vi "Transcriptor LabVIEW to C code 1.vi"(8 "error in (no error)":errorcluster, 9 "nested level":i32, 10 "GObject stop":refnum<vi>, 11 "GObject start":refnum<vi>) -> (0 "error out":errorcluster, 3 "Transcripted code":string)   [LabVIEW 2014]
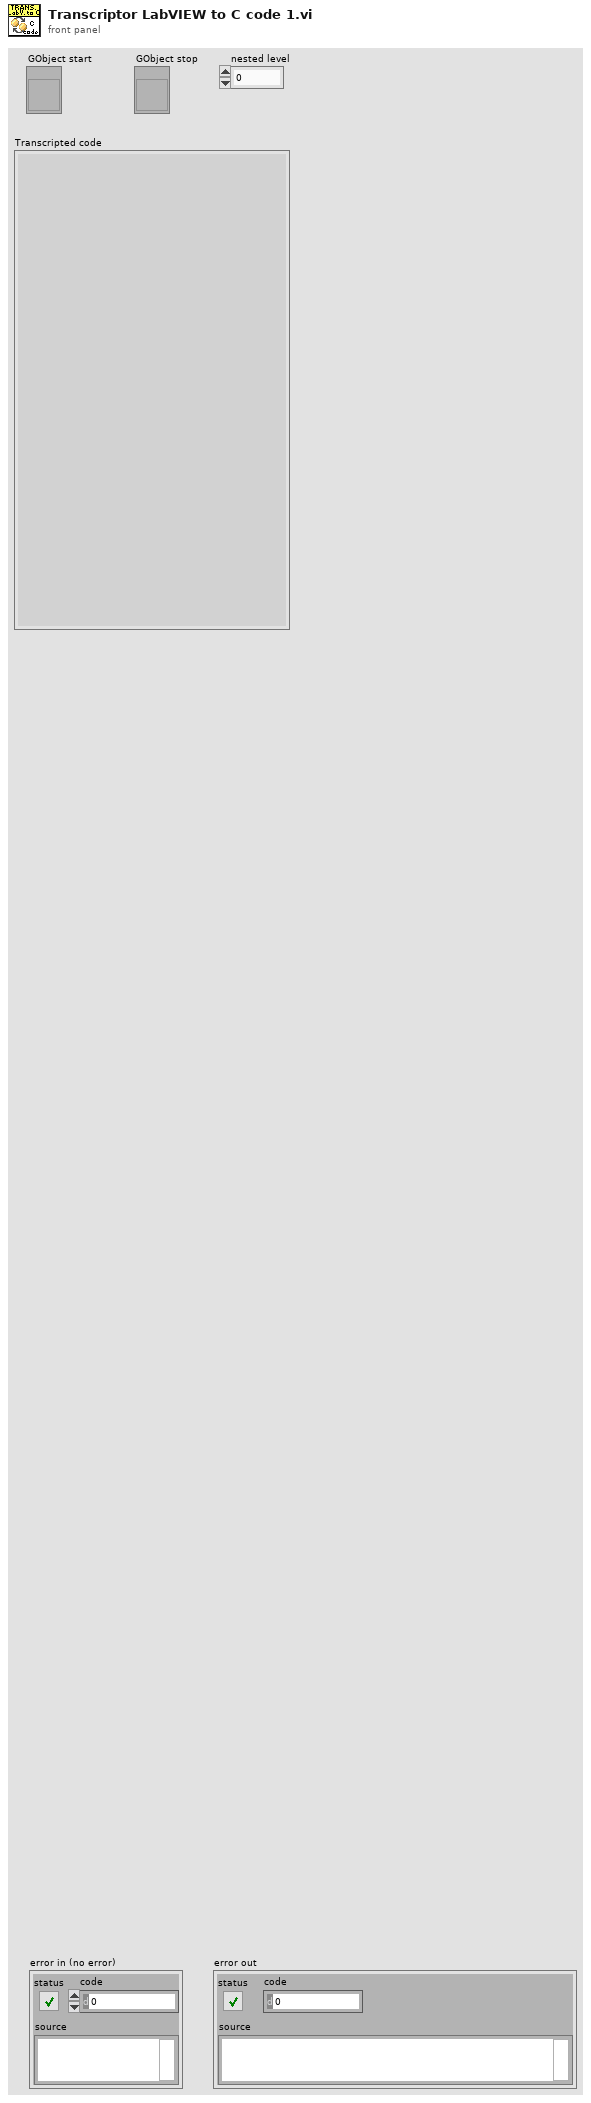
[diagram p1: front panel]
types:
  T1 = cluster{"transcripted code":string[], "element translation order":string[]}
  T2 = cluster{"terminals datatypes":string[][], "terminal\nconnected?":bool[], "terminal captions":string[], "term. count":i32, "terminal\nIsSource?":bool[], "SubVI name":string, "connected\nwires refs.":refnum<vi>[], "coerced\ndot?":bool[], "terminals[]":refnum<vi>[]}
  T3 = cluster{"terminals datatypes":string[][], "terminal\nconnected?":bool[], "terminal captions":string[], "term. count":i32, "terminal\nIsSource?":bool[], "SubVI name":string, "connected\nwires refs.":refnum<vi>[], "coerced dot?":bool[], "terminals[]":refnum<vi>[]}
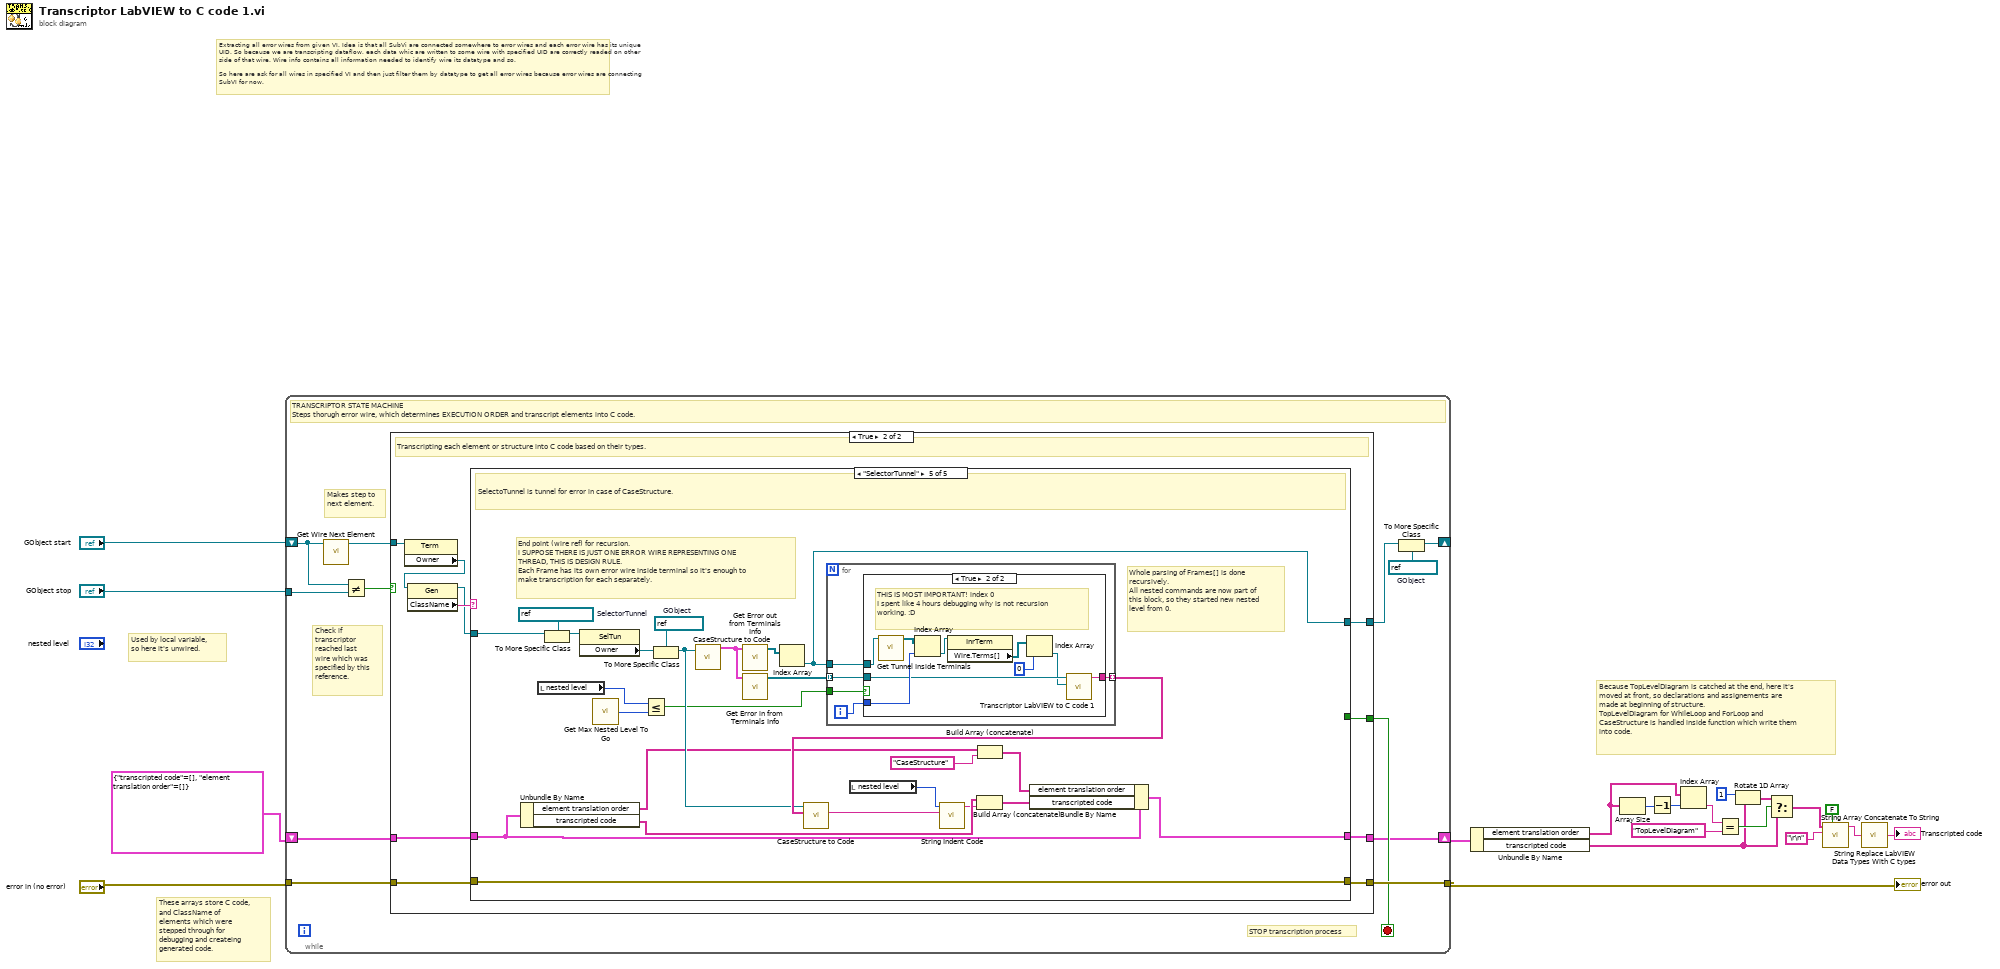
[diagram p0: block diagram]
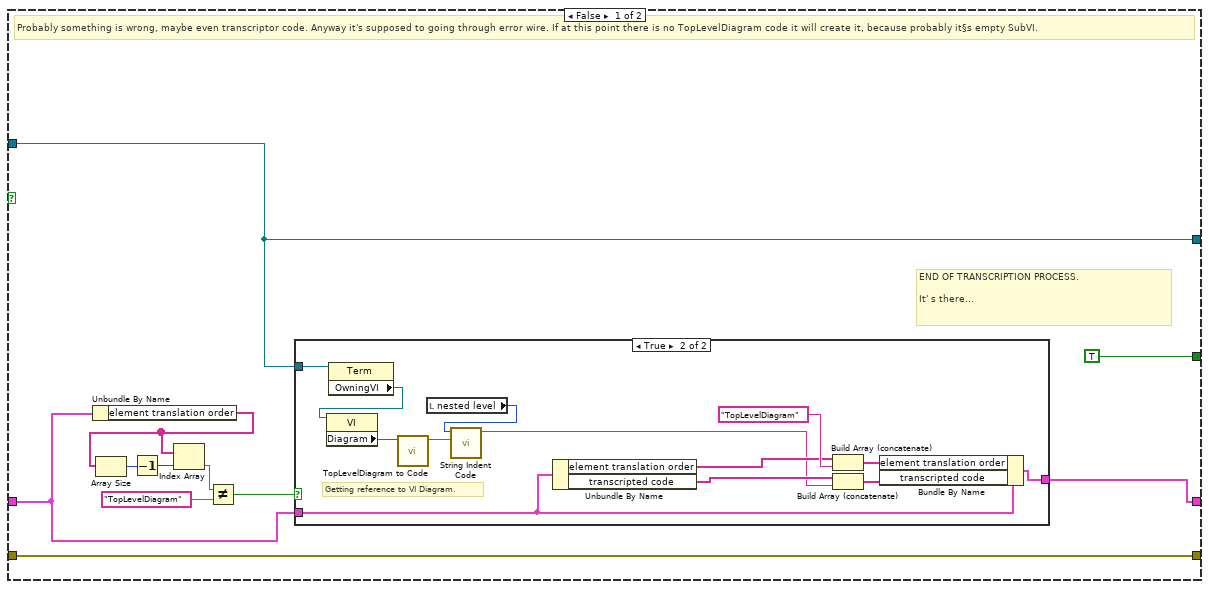
[diagram p2: hidden frame]
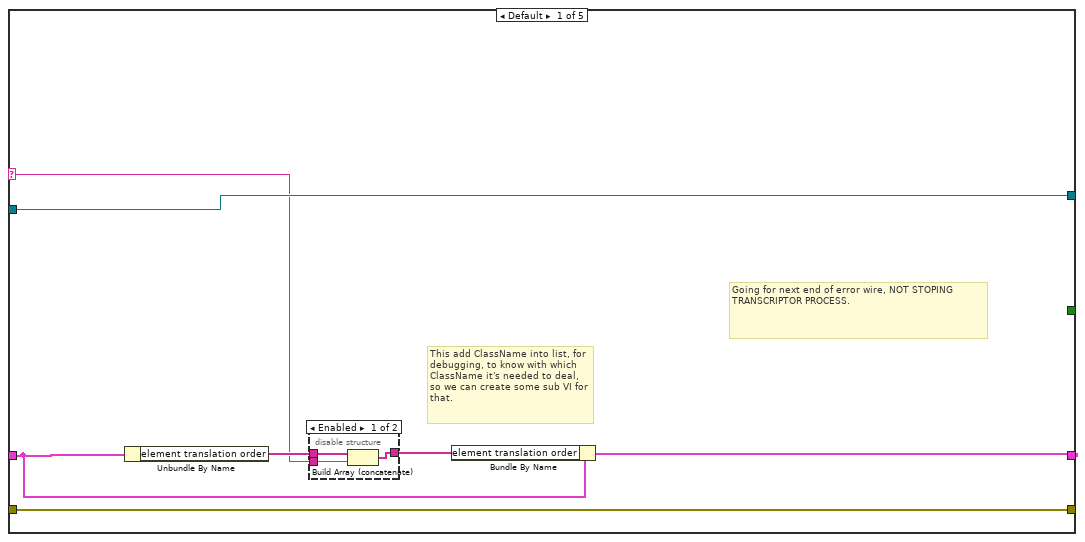
[diagram p4: hidden frame]
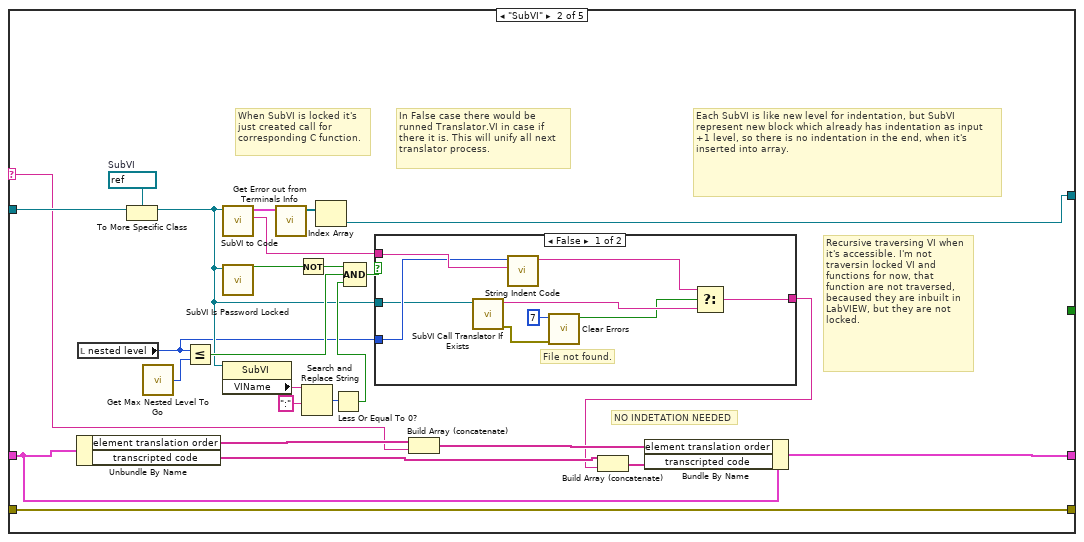
[diagram p6: hidden frame]
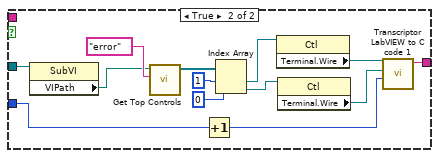
[diagram p7: hidden frame]
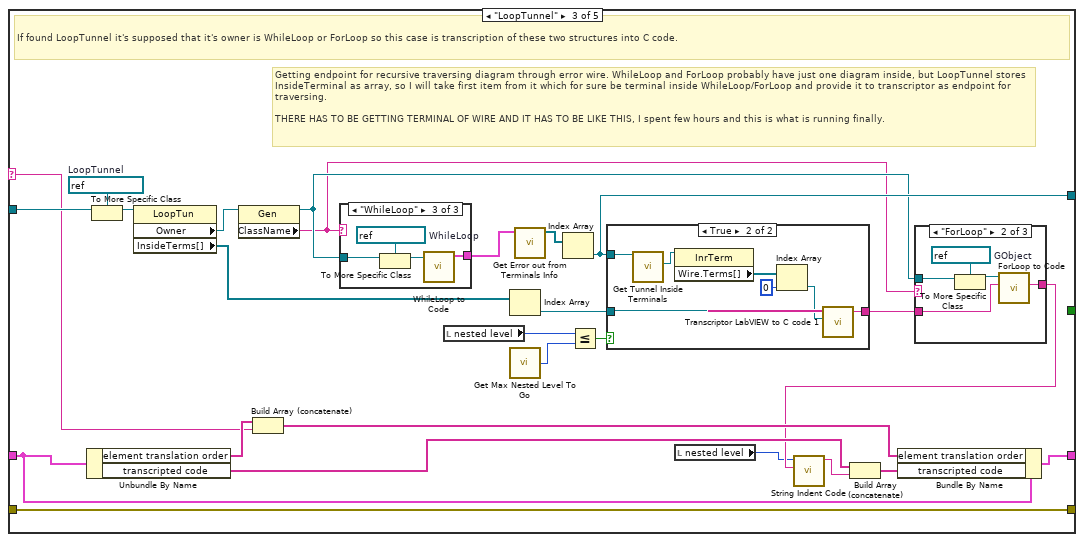
[diagram p8: hidden frame]
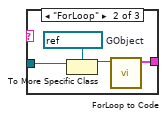
[diagram p10: hidden frame]
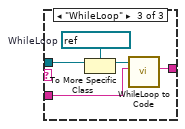
[diagram p12: hidden frame]
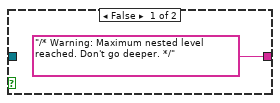
[diagram p13: hidden frame]
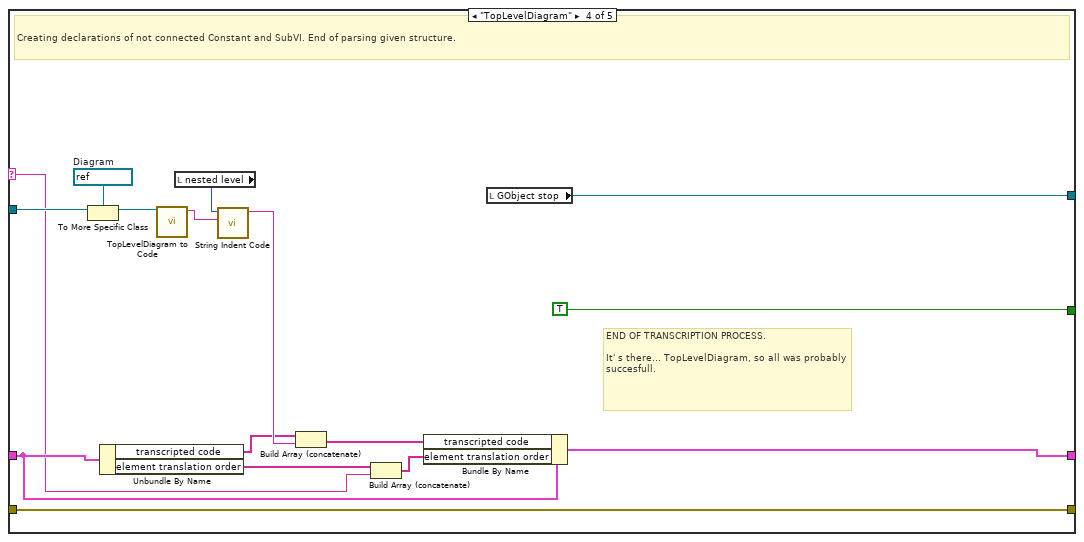
[diagram p14: hidden frame]
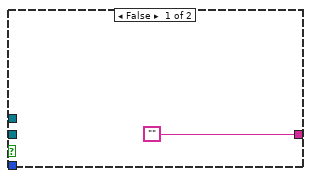
[diagram p15: hidden frame]
diagram:
  # "Because TopLevelDiagram is catched at the end, here it's moved at front, so declarations and assignements are made at beginning of structure.\nTopLevelDiagram for WhileLoop and ForLoop and CaseStructure is handled inside function which write them into code."
  # "Used by local variable, so here it's unwired."
  # "These arrays store C code, and ClassName of elements which were stepped through for debugging and createing generated code."
  # "Extracting all error wires from given VI. Idea is that all SubVi are connected somewhere to error wires and each error wire has its unique UID. So because we are transcripting dataflow, each data whic are written to some wire with specified UID are correctly readed on other side of that wire. Wire info contains all information needed to identify wire its datatype and so.\n\nSo here are ask for all wires in specified VI and then just filter them by datatype to get all error wires because error wires are connecting SubVI for now."
  n1 = while {
    tunnel: [w31] -> w15
    tunnel: "error in (no error)" -> [w30]
    shift-right: [w26] -> _
    shift-left: "GObject start" -> [w22]
    tunnel: "GObject stop" -> [w21]
    shift-right: [w24] -> w16
    shift-left: T1 {"transcripted code"=[], "element translation order"=[]} -> [w25]
    stop <- w29 stop-if-true
    w28 = refnum<vi> refnum  # GObject
    # "Makes step to next element."
    # "Check if transcriptor reached last wire which was specified by this reference."
    # "STOP transcription process"
    # "TRANSCRIPTOR STATE MACHINE\nSteps thorugh error wire, which determines EXECUTION ORDER and transcript elements into C code."
    n2 = call "Get Wire Next Element.vi"("start object"=w22) -> ("next terminal"=w32:refnum<vi>)  [unwired: 9 in, 1 out]
    n3 = Not Equal?(x=w22, y=w21) -> (x != y?=w23:bool)
    n4 = case shown="True" w23 {
      tunnel: w32 -> [w35 w63]
      tunnel: [w43 w67] -> w31
      tunnel: w30 -> [w43 w66]
      tunnel: [w35 w65] -> w27
      tunnel: [TRUE w64] -> w29
      tunnel: w25 -> [w34 w62]
      tunnel: [w33 w61] -> w24
      frame False {
        # "END OF TRANSCRIPTION PROCESS.\n\nIt' s there..."
        # "Probably something is wrong, maybe even transcriptor code. Anyway it's supposed to going through error wire. If at this point there is no TopLevelDiagram code it will create it, because probably it§s empty SubVI."
        n5 = Unbundle By Name(w34) -> ("element translation order"=w41:string[])
        n6 = Array Size(array=w41) -> (size(s)=w40:i32)
        n7 = Decrement(x=w40) -> (x-1=w39:i32)
        n8 = Index Array(array=w41, index=w39) -> (element=w38:string)
        n9 = Not Equal?(x=w38, y="TopLevelDiagram") -> (x != y?=w36:bool)
        n10 = case shown="True" w36 {
          tunnel: w35 -> [_ w57]
          tunnel: w34 -> [w44 w51]
          tunnel: [w44 w52] -> w33
          frame False {
          }
          frame True {
            # "Getting reference to VI Diagram."
            n11 = property class="Term"(reference=w57) -> ("OwningVI"=w54:refnum<vi>)  [unwired: 1 in, 2 out]
            n12 = property class="VI"(reference=w54) -> ("Diagram"=w53:refnum<vi>)  [unwired: 1 in, 2 out]
            n13 = call "TopLevelDiagram to Code.vi"("Diagram ref"=w53) -> ("transcripted code"=w55:string)  [unwired: 10 in]
            n14 = local read "nested level"() -> (w56:i32)
            n15 = call "String Indent Code.vi"("complete code"=w55, "actual nested level"=w56) -> ("indented code"=w45:string)  [unwired: 9 in]
            n16 = Unbundle By Name(w51) -> ("element translation order"=w48:string[], "transcripted code"=w47:string[])
            n17 = Build Array (concatenate)(w48, "TopLevelDiagram" ("y")) -> (w49:string[])
            n18 = Build Array (concatenate)(w47, w45) -> (w46:string[])
            n19 = Bundle By Name(cluster=w51, "element translation order"=w49, "transcripted code"=w46) -> (w52:T1)
          }
        }
      }
      frame True {
        # "Transcripting each element or structure into C code based on their types."
        n20 = property class="Term"(reference=w63) -> ("Owner"=w59:refnum<vi>)  [unwired: 1 in, 2 out]
        n21 = property class="Gen"(reference=w59) -> (reference out=w58:refnum<vi>, "ClassName"=w60:string)  [unwired: 1 in, 1 out]
        n22 = case shown="\"SelectorTunnel\"" w60 {
          selector: w60 -> [w68 w79 w127 w179 _]
          tunnel: w58 -> [w73 w93 w151 w186 w216]
          tunnel: [w74 w103 w149 w194 w218] -> w67
          tunnel: w66 -> [w74 w103 w149 w194 w218]
          tunnel: [w73 w94 w144 w188 w208] -> w65
          tunnel: [_ _ _ TRUE _] -> w64
          tunnel: w62 -> [w71 w100 w142 w191 w203]
          tunnel: [w69 w99 w141 w190 w204] -> w61
          frame Default {
            # "Going for next end of error wire, NOT STOPING TRANSCRIPTOR PROCESS."
            # "This add ClassName into list, for debugging, to know with which ClassName it's needed to deal, so we can create some sub VI for that."
            n23 = Unbundle By Name(w71) -> ("element translation order"=w72:string[])
            n24 = disable-structure shown="Enabled" {
              disable-tunnel: w72 -> [w77 w78]
              disable-tunnel: w68 -> [w76 _]
              disable-tunnel: [w75 w78] -> w70
              frame Enabled {
                n25 = Build Array (concatenate)(w77, w76) -> (w75:string[])
              }
              frame Disabled {
              }
            }
            n26 = Bundle By Name(cluster=w71, "element translation order"=w70) -> (w69:T1)
          }
          frame "SubVI" {
            w104 = refnum<vi> refnum  # SubVI
            # "In False case there would be runned Translator.VI in case if there it is. This will unify all next translator process."
            # "When SubVI is locked it's just created call for corresponding C function."
            # "NO INDETATION NEEDED"
            # "Each SubVI is like new level for indentation, but SubVI represent new block which already has indentation as input +1 level, so there is no indentation in the end, when it's inserted into array."
            # "Recursive traversing VI when it's accessible. I'm not traversin locked VI and\nfunctions for now, that function are not traversed, becaused they are inbuilt in LabVIEW, but they are not locked."
            n27 = Unbundle By Name(w100) -> ("element translation order"=w96:string[], "transcripted code"=w97:string[])
            n28 = local read "nested level"() -> (w81:i32)
            n29 = To More Specific Class(target class=w104, reference=w93) -> (specific class reference=w83:refnum<vi>)  [unwired: 1 in, 1 out]
            n30 = call "Get Max Nested Level To Go.vi"() -> ("max nested level"=w82:i32)
            n31 = Less Or Equal?(x=w81, y=w82) -> (x <= y?=w90:bool)
            n32 = call "SubVI to Code.vi"("reference"=w83) -> ("C code"=w92:string, "SubVI terminals info"=w101:T2)  [unwired: 9 in]
            n33 = call "SubVI Is Password Locked.vi"("SubVI ref"=w83) -> ("isPasswordLocked?"=w89:bool)  [unwired: 9 in, 1 out]
            n34 = property class="SubVI"(reference=w83) -> ("VIName"=w87:string)  [unwired: 1 in, 2 out]
            n35 = call "Get Error out from Terminals Info.vi"("terminals info"=w101) -> ("error out terminals"=w102:refnum<vi>[])  [unwired: 9 in, 1 out]
            n36 = Not(x=w89) -> (.not. x?=w88:bool)
            n37 = Search and Replace String(input string=w87, search string=":") -> (number of replacements=w85:i32)  [unwired: 6 in, 3 out]
            n38 = Index Array(array=w102) -> (element=w94:refnum<vi>)  [unwired: 1 in]
            n39 = Less Or Equal To 0?(x=w85) -> (x <= 0?=w84:bool)
            n40 = Compound Arithmetic op=AND(w88, w90, w84) -> (w91:bool)
            n41 = case shown="False" w91 {
              tunnel: w83 -> [w110 w126]
              tunnel: [w112 w125] -> w80
              tunnel: w92 -> [w113 _]
              tunnel: w81 -> [w111 w124]
              frame False {
                # "File not found."
                n42 = call "SubVI Call Translator If Exists.vi"("SubVI Refnum"=w110) -> ("Error Out"=w109:errorcluster, "Replaced Code"=w107:string)  [unwired: 9 in]
                n43 = call "String Indent Code.vi"("complete code"=w113, "actual nested level"=w111) -> ("indented code"=w105:string)  [unwired: 9 in]
                n44 = call <vilib>:"Clear Errors.vi"("error in (no error)"=w109, "specific error code to clear (0: all)"=7) -> ("specific error cleared?"=w106:bool)  [unwired: 4 in, 1 out]
                n45 = Select(t=w105, s=w106, f=w107) -> (s? t:f=w112:string)
              }
              frame True {
                n46 = property class="SubVI"(reference=w126) -> ("VIPath"=w119:path)  [unwired: 1 in, 2 out]
                n47 = call "Get Top Controls.vi"("DataType"="error", "vi path"=w119) -> ("Controls Referencies Array"=w122:refnum<vi>[])  [unwired: 8 in, 1 out]
                n48 = Increment(x=w124) -> (x+1=w114:i32)
                n49 = Index Array(array=w122, index #1=1 ("index"), index #2=0 ("index")) -> (element #1=w118:refnum<vi>, element #2=w117:refnum<vi>)
                n50 = property on="Property Node" class="Ctl"(reference=w118) -> ("Terminal.Wire"=w116:refnum<vi>)  [unwired: 1 in, 2 out]
                n51 = property on="Property Node" class="Ctl"(reference=w117) -> ("Terminal.Wire"=w115:refnum<vi>)  [unwired: 1 in, 2 out]
                n52 = call "Transcriptor LabVIEW to C code 1.vi"("nested level"=w114, "GObject stop"=w115, "GObject start"=w116) -> ("Transcripted code"=w125:string)  [unwired: 7 in, 1 out]
              }
            }
            n53 = Build Array (concatenate)(w96, w79) -> (w95:string[])
            n54 = Build Array (concatenate)(w97, w80) -> (w98:string[])
            n55 = Bundle By Name(cluster=w100, "element translation order"=w95, "transcripted code"=w98) -> (w99:T1)
          }
          frame "LoopTunnel" {
            w152 = refnum<vi> refnum  # LoopTunnel
            # "Getting endpoint for recursive traversing diagram through error wire. WhileLoop and ForLoop probably have just one diagram inside, but LoopTunnel stores InsideTerminal as array, so I will take first item from it which for sure be terminal inside WhileLoop/ForLoop and provide it to transcriptor as endpoint for traversing.\n\nTHERE HAS TO BE GETTING TERMINAL OF WIRE AND IT HAS TO BE LIKE THIS, I spent few hours and this is what is running finally."
            # "If found LoopTunnel it's supposed that it's owner is WhileLoop or ForLoop so this case is transcription of these two structures into C code."
            n56 = Unbundle By Name(w142) -> ("element translation order"=w136:string[], "transcripted code"=w140:string[])
            n57 = To More Specific Class(target class=w152, reference=w151) -> (specific class reference=w150:refnum<vi>)  [unwired: 1 in, 1 out]
            n58 = property class="LoopTun"(reference=w150) -> ("Owner"=w138:refnum<vi>, "InsideTerms[]"=w148:refnum<vi>[])  [unwired: 1 in, 2 out]
            n59 = property class="Gen"(reference=w138) -> (reference out=w130:refnum<vi>, "ClassName"=w129:string)  [unwired: 1 in, 1 out]
            n60 = Build Array (concatenate)(w136, w127) -> (w135:string[])
            n61 = case shown="\"WhileLoop\"" w129 {
              tunnel: [_ w155 w159] -> w137
              tunnel: w130 -> [_ w153 w158]
              frame Default {
                # "For now there is implemented:\n+ ForLoop\n+ WhileLoop"
              }
              frame "ForLoop" {
                w156 = refnum<vi> refnum  # GObject
                n62 = To More Specific Class(target class=w156, reference=w153) -> (specific class reference=w154:refnum<vi>)  [unwired: 1 in, 1 out]
                n63 = call "ForLoop to Code.vi"("GObj Refnum"=w154) -> ("terminals info"=w155:T3)  [unwired: 8 in, 2 out]
              }
              frame "WhileLoop" {
                w160 = refnum<vi> refnum  # WhileLoop
                n64 = To More Specific Class(target class=w160, reference=w158) -> (specific class reference=w157:refnum<vi>)  [unwired: 1 in, 1 out]
                n65 = call "WhileLoop to Code.vi"("WhileLoop ref"=w157) -> ("terminals info"=w159:T3)  [unwired: 8 in, 2 out]
              }
            }
            n66 = local read "nested level"() -> (w145:i32)
            n67 = Index Array(array=w148) -> (element=w147:refnum<vi>)  [unwired: 1 in]
            n68 = call "Get Max Nested Level To Go.vi"() -> ("max nested level"=w131:i32)
            n69 = call "Get Error out from Terminals Info.vi"("terminals info"=w137) -> ("error out terminals"=w146:refnum<vi>[])  [unwired: 9 in, 1 out]
            n70 = Index Array(array=w146) -> (element=w144:refnum<vi>)  [unwired: 1 in]
            n71 = Less Or Equal?(x=w145, y=w131) -> (x <= y?=w143:bool)
            n72 = case shown="True" w143 {
              tunnel: w147 -> [_ w177]
              tunnel: w144 -> [_ w174]
              tunnel: ["/* Warning: Maximum nested level reached. Don't go deeper. */" ("Transcripted code") w178] -> w139
              frame False {
              }
              frame True {
                n73 = call "Get Tunnel Inside Terminals.vi"("Terminal in"=w174) -> ("Terms[0]"=w172:refnum<vi>)  [unwired: 9 in, 1 out]
                n74 = property class="InrTerm"(reference=w172) -> ("Wire.Terms[]"=w176:refnum<vi>[])  [unwired: 1 in, 2 out]
                n75 = Index Array(array=w176, index=0) -> (element=w173:refnum<vi>)
                n76 = call "Transcriptor LabVIEW to C code 1.vi"("GObject stop"=w173, "GObject start"=w177) -> ("Transcripted code"=w178:string)  [unwired: 8 in, 1 out]
              }
            }
            n77 = local read "nested level"() -> (w132:i32)
            n78 = case shown="\"ForLoop\"" w129 {
              tunnel: [_ w161 w166] -> w133
              tunnel: w130 -> [_ w163 w169]
              tunnel: w139 -> [_ w162 w167]
              frame Default {
                # "For now there is implemented:\n+ ForLoop\n+ WhileLoop"
              }
              frame "ForLoop" {
                w165 = refnum<vi> refnum  # GObject
                n79 = To More Specific Class(target class=w165, reference=w163) -> (specific class reference=w164:refnum<vi>)  [unwired: 1 in, 1 out]
                n80 = call "ForLoop to Code.vi"("C code in"=w162, "GObj Refnum"=w164) -> ("C code"=w161:string)  [unwired: 7 in, 2 out]
              }
              frame "WhileLoop" {
                w170 = refnum<vi> refnum  # WhileLoop
                n81 = To More Specific Class(target class=w170, reference=w169) -> (specific class reference=w168:refnum<vi>)  [unwired: 1 in, 1 out]
                n82 = call "WhileLoop to Code.vi"("C code in"=w167, "WhileLoop ref"=w168) -> ("C code"=w166:string)  [unwired: 7 in, 2 out]
              }
            }
            n83 = call "String Indent Code.vi"("complete code"=w133, "actual nested level"=w132) -> ("indented code"=w134:string)  [unwired: 9 in]
            n84 = Build Array (concatenate)(w140, w134) -> (w128:string[])
            n85 = Bundle By Name(cluster=w142, "element translation order"=w135, "transcripted code"=w128) -> (w141:T1)
          }
          frame "TopLevelDiagram" {
            w185 = refnum<vi> refnum  # Diagram
            # "END OF TRANSCRIPTION PROCESS.\n\nIt' s there... TopLevelDiagram, so all was probably succesfull."
            # "Creating declarations of not connected Constant and SubVI. End of parsing given structure."
            n86 = To More Specific Class(target class=w185, reference=w186) -> (specific class reference=w187:refnum<vi>)  [unwired: 1 in, 1 out]
            n87 = Unbundle By Name(w191) -> ("transcripted code"=w180:string[], "element translation order"=w192:string[])
            n88 = call "TopLevelDiagram to Code.vi"("Diagram ref"=w187) -> ("transcripted code"=w184:string)  [unwired: 10 in]
            n89 = local read "nested level"() -> (w182:i32)
            n90 = call "String Indent Code.vi"("complete code"=w184, "actual nested level"=w182) -> ("indented code"=w183:string)  [unwired: 9 in]
            n91 = Build Array (concatenate)(w180, w183) -> (w181:string[])
            n92 = Build Array (concatenate)(w192, w179) -> (w189:string[])
            n93 = Bundle By Name(cluster=w191, "transcripted code"=w181, "element translation order"=w189) -> (w190:T1)
            n94 = local read "GObject stop"() -> (w188:refnum<vi>)
          }
          frame "SelectorTunnel" {
            w213 = refnum<vi> refnum  # GObject
            w217 = refnum<vi> refnum  # SelectorTunnel
            # "End point (wire ref) for recursion.\ni SUPPOSE THERE IS JUST ONE ERROR WIRE REPRESENTING ONE THREAD, THIS IS DESIGN RULE.\nEach Frame has its own error wire inside terminal so it's enough to make transcription for each separately."
            # "Whole parsing of Frames[] is done recursively.\nAll nested commands are now part of this block, so they started new nested level from 0."
            # "SelectoTunnel is tunnel for error in case of CaseStructure."
            n95 = Unbundle By Name(w203) -> ("element translation order"=w200:string[], "transcripted code"=w205:string[])
            n96 = local read "nested level"() -> (w206:i32)
            n97 = To More Specific Class(target class=w217, reference=w216) -> (specific class reference=w215:refnum<vi>)  [unwired: 1 in, 1 out]
            n98 = property class="SelTun"(reference=w215) -> ("Owner"=w214:refnum<vi>)  [unwired: 1 in, 2 out]
            n99 = call "Get Max Nested Level To Go.vi"() -> ("max nested level"=w198:i32)
            n100 = Less Or Equal?(x=w206, y=w198) -> (x <= y?=w202:bool)
            n101 = To More Specific Class(target class=w213, reference=w214) -> (specific class reference=w209:refnum<vi>)  [unwired: 1 in, 1 out]
            n102 = call "CaseStructure to Code.vi"("case struct ref."=w209) -> ("terminals info"=w211:T3)  [unwired: 8 in, 2 out]
            n103 = call "Get Error out from Terminals Info.vi"("terminals info"=w211) -> ("error out terminals"=w219:refnum<vi>[])  [unwired: 9 in, 1 out]
            n104 = call "Get Error in from Terminals Info.vi"("terminals info"=w211) -> ("error in terminals[]"=w207:refnum<vi>[])  [unwired: 9 in, 1 out]
            n105 = Index Array(array=w219) -> (element=w208:refnum<vi>)  [unwired: 1 in]
            n106 = for {
              tunnel: [w224] -> w210 mode=indexing
              tunnel: w202 -> [w223]
              tunnel: w208 -> [w222]
              tunnel: w207 -> [w221] mode=indexing
              i -> [w220]
              n107 = case shown="True" w223 {
                tunnel: ["" w234] -> w224
                tunnel: w222 -> [_ w227]
                tunnel: w221 -> [_ w232]
                tunnel: w220 -> [_ w233]
                frame False {
                }
                frame True {
                  # "THIS IS MOST IMPORTANT! index 0\nI spent like 4 hours debugging why is not recursion working. :D"
                  n108 = call "Get Tunnel Inside Terminals.vi"("Terminal in"=w227) -> ("InsideTerms[]"=w226:refnum<vi>[])  [unwired: 9 in, 1 out]
                  n109 = Index Array(array=w226, index=w233) -> (element=w228:refnum<vi>)
                  n110 = property class="InrTerm"(reference=w228) -> ("Wire.Terms[]"=w231:refnum<vi>[])  [unwired: 1 in, 2 out]
                  n111 = Index Array(array=w231, index=0) -> (element=w229:refnum<vi>)
                  n112 = call "Transcriptor LabVIEW to C code 1.vi"("GObject stop"=w229, "GObject start"=w232) -> ("Transcripted code"=w234:string)  [unwired: 8 in, 1 out]
                }
              }
            }
            n113 = call "CaseStructure to Code.vi"("Frames code[]"=w210, "case struct ref."=w209) -> ("C code"=w199:string)  [unwired: 7 in, 2 out]
            n114 = local read "nested level"() -> (w196:i32)
            n115 = call "String Indent Code.vi"("complete code"=w199, "actual nested level"=w196) -> ("indented code"=w201:string)  [unwired: 9 in]
            n116 = Build Array (concatenate)(w205, w201) -> (w195:string[])
            n117 = Build Array (concatenate)(w200, "CaseStructure") -> (w197:string[])
            n118 = Bundle By Name(cluster=w203, "element translation order"=w197, "transcripted code"=w195) -> (w204:T1)
          }
        }
      }
    }
    n119 = To More Specific Class(target class=w28, reference=w27) -> (specific class reference=w26:refnum<vi>)  [unwired: 1 in, 1 out]
  }
  "error out" <- w15
  n120 = Unbundle By Name(w16) -> ("element translation order"=w3:string[], "transcripted code"=w4:string[])
  n121 = Array Size(array=w3) -> (size(s)=w12:i32)
  n122 = Decrement(x=w12) -> (x-1=w11:i32)
  n123 = Index Array(array=w3, index=w11) -> (element=w10:string)
  n124 = Equal?(x=w10, y="TopLevelDiagram") -> (x = y?=w7:bool)
  n125 = Rotate 1D Array(1:w4, 2:1 ("n")) -> (0:w6:string[])
  n126 = Select(t=w6, s=w7, f=w4) -> (s? t:f=w5:string[])
  n127 = call "String Array Concatenate To String.vi"("insert last delimiter?"=FALSE, "Delimiter char"="\r\n", "Array String In"=w5) -> ("String"=w14:string)  [unwired: 8 in]
  n128 = call "String Replace LabVIEW Data Types With C types.vi"("C code"=w14) -> ("C code, replaced datatypes"=→"Transcripted code":string)
